vi "Compute Process Data.vi"(0 "Acquisition mode":T1, 5 "Processing loop variables":T3 {"CurrInverter"."last updated" format="%<%H:%M\n%d/%m/%Y>T"; "CurrInverter"."set flag" items=["False", "True"]}, 7 "InverterWaveforms":T11, 9 "ESR scaling":T10[](array[typedef]), 11 "error in (no error)":errorcluster, 12 "Use dummy Vout?":bool, 13 "Dummy Vrms":dbl=120.0, 14 "reset averaging":bool) -> (4 "DataProcAuxData":T2[](array[typedef]), 6 "Processing loop vars out":T3 {"CurrInverter"."last updated" format="%<%H:%M\n%d/%m/%Y>T"; "CurrInverter"."set flag" items=["False", "True"]}, 8 "Max ESR":dbl[](array[numeric]), 15 "error out":errorcluster)   [LabVIEW 2019, in "Main.lvclass"]
doc: "Developed by Kevin Thompson\nkevin@thompsonengineering.net\n\nCopyright 2020\nThompson Engineering, LLC"
uses:
  Main.lvclass
  subvis/DataTypes/Processing loop variables--cluster.ctl
  subvis/DataTypes/averaging variables.ctl
  subvis/DataTypes/ESR alarm variables.ctl
  Common/DataTypes/Inverter database record v2--cluster.ctl
  Common/DataTypes/inverter info v2--cluster.ctl
  Common/DataTypes/inverter gain range--cluster.ctl
  Common/DataTypes/inverter offset range--cluster.ctl
  Common/DataTypes/InverterWaveforms--cluster.ctl
  Common/DataTypes/ChannelWaveforms--cluster.ctl
  subvis/DataTypes/ESR scaling--cluster.ctl
  DataTypes/DataProcessAuxData--cluster.ctl
  Common/DataTypes/Acquisition Mode--cluster.ctl
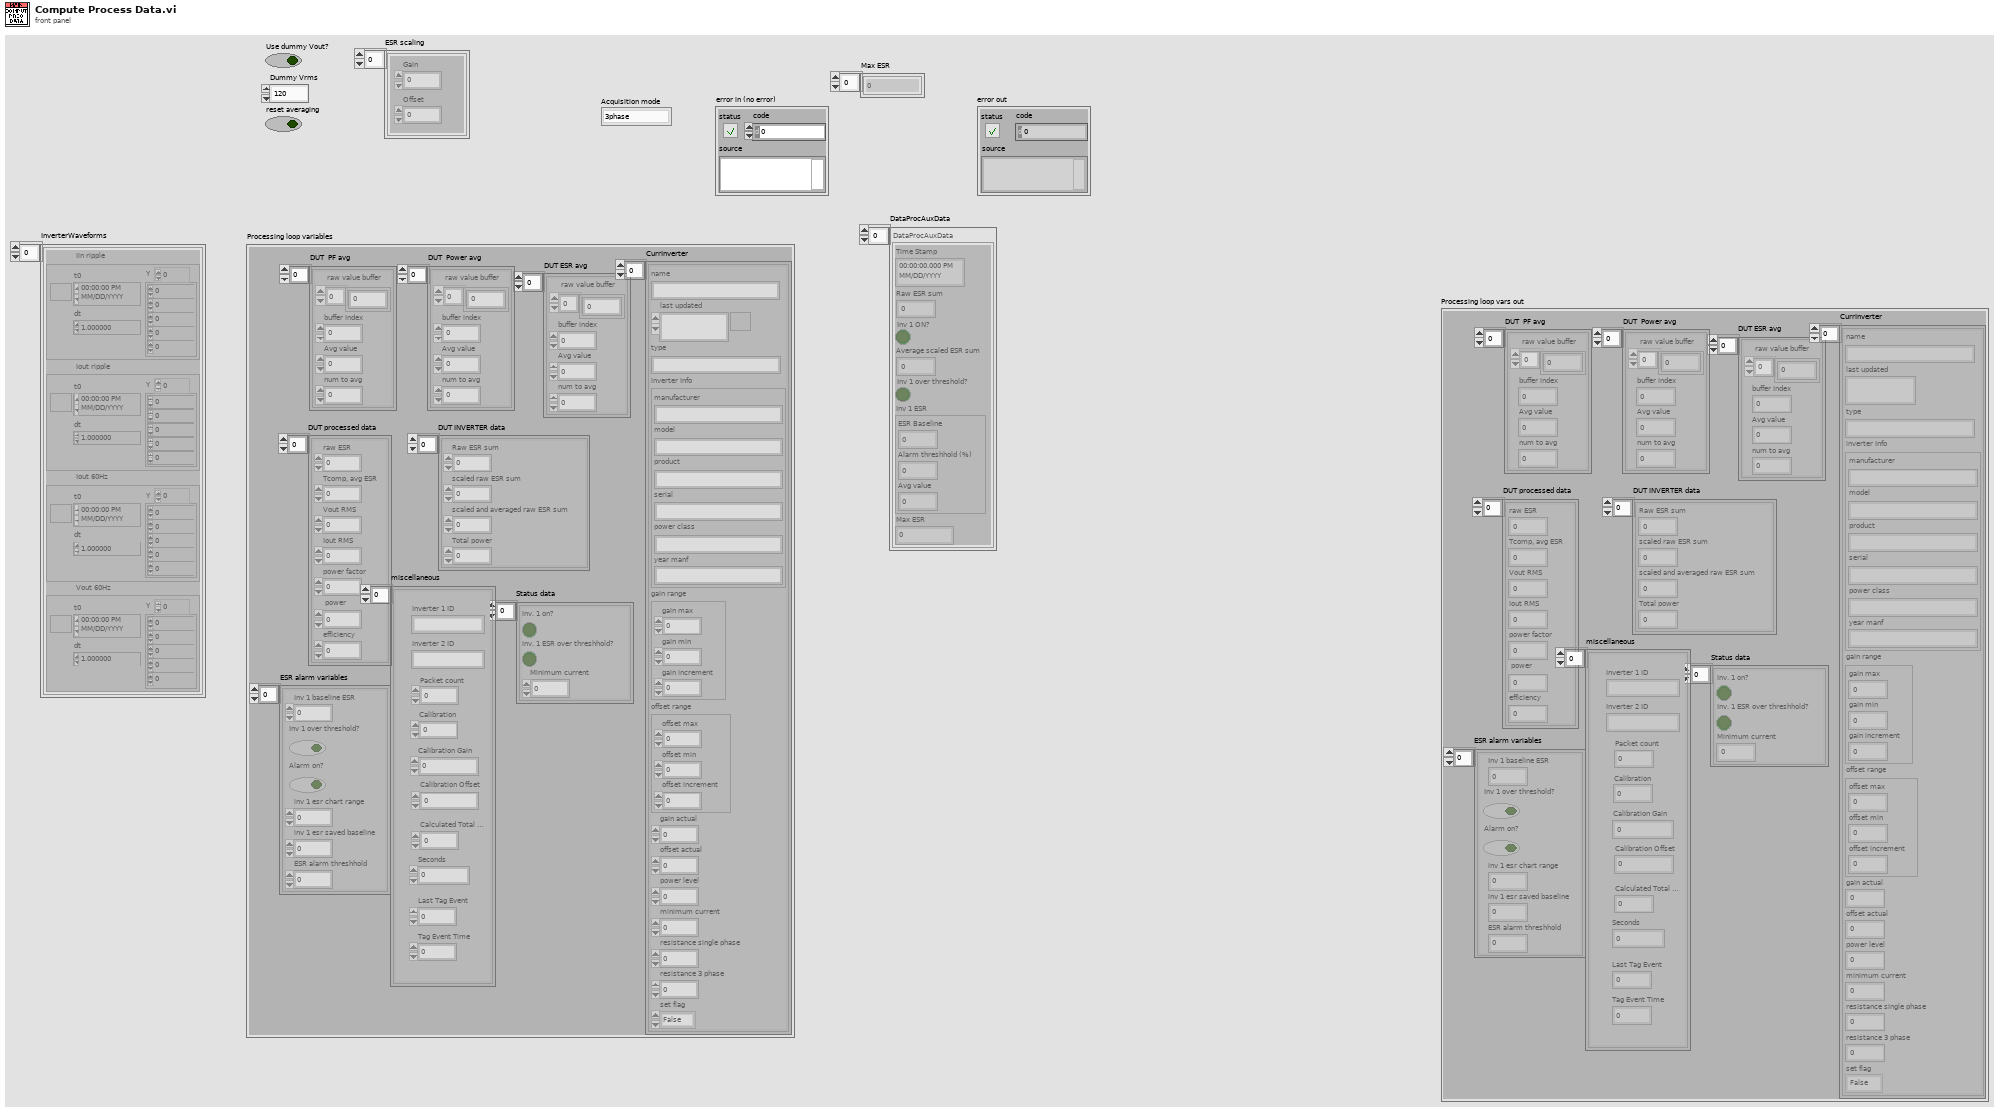
[diagram p1: front panel]
types:
  T1 = typedef "Acquisition Mode--cluster.ctl" = enum16{"3phase", "Single"}
  T2 = typedef "DataProcessAuxData--cluster.ctl" = cluster{"Time Stamp":timestamp, "Raw ESR sum":dbl, "Inv 1 ON?":bool, "Average scaled ESR sum":dbl, "Inv 1 over threshold?":bool, "Inv 1 ESR":cluster{"ESR Baseline":dbl, "Alarm threshhold (%)":dbl, "Avg value":dbl}, "Max ESR":dbl}
  T3 = typedef "Main.lvclass/Processing loop variables--cluster.ctl" = cluster{"DUT ESR avg":T4[], "DUT  PF avg":T4[], "DUT  Power avg ":T4[], "DUT processed data":cluster{"raw ESR":dbl, "Tcomp, avg ESR":dbl, "Vout RMS":dbl, "Iout RMS":dbl, "power factor":dbl, "power":dbl, "efficiency":dbl}[], "ESR alarm variables":T5[], "Status data":cluster{"Inv. 1 on?":bool, "Inv. 1 ESR over threshhold?":bool, "Minimum current":dbl}[], "CurrInverter":T6[], "miscellaneous":cluster{"Inverter 1 ID":string, "Inverter 2 ID":string, "Packet count":u32, "Calibration":dbl, "Calibration Gain":dbl, "Calibration Offset":dbl, "Calculated Total Power":dbl, "Seconds":dbl, "Last Tag Event":dbl, "Tag Event Time":dbl}[], "DUT INVERTER data":cluster{"Raw ESR sum":dbl, "scaled raw ESR sum":dbl, "scaled and averaged raw ESR sum":dbl, "Total power":dbl}[]}
  T4 = typedef "Main.lvclass/averaging variables.ctl" = cluster{"raw value buffer":dbl[], "buffer index":i32, "Avg value":dbl, "num to avg":i32}
  T5 = typedef "Main.lvclass/ESR alarm variables.ctl" = cluster{"Inv 1 baseline ESR":dbl, "Inv 1 over threshold?":bool, "Alarm on?":bool, "inv 1 esr chart range":dbl, "inv 1 esr saved baseline":dbl, "ESR alarm threshhold":dbl}
  T6 = typedef "Inverter database record v2--cluster.ctl" = cluster{"name":string, "last updated":timestamp, "type":string, "inverter Info":T7, "gain range":T8, "offset range":T9, "gain actual":dbl, "offset actual":dbl, "power level":dbl, "minimum current":dbl, "resistance single phase":dbl, "resistance 3 phase":dbl, "set flag":u16}
  T7 = typedef "inverter info v2--cluster.ctl" = cluster{"manufacturer":string, "model":string, "product":string, "serial":string, "power class":string, "year manf":string}
  T8 = typedef "inverter gain range--cluster.ctl" = cluster{"gain max":dbl, "gain min":dbl, "gain increment":dbl}
  T9 = typedef "inverter offset range--cluster.ctl" = cluster{"offset max":dbl, "offset min":dbl, "offset increment":dbl}
  T10 = typedef "Main.lvclass/ESR scaling--cluster.ctl" = cluster{"Gain":dbl, "Offset":dbl}
  T11 = typedef "InverterWaveforms--cluster.ctl" = T12[]
  T12 = typedef "ChannelWaveforms--cluster.ctl" = cluster{"Iin ripple ":waveform(dbl), "Iout ripple ":waveform(dbl), "Iout 60Hz":waveform(dbl), "Vout 60Hz":waveform(dbl)}
  T13 = cluster{"ESR Baseline":dbl, "Alarm threshhold (%)":dbl, "Avg value":dbl}[]
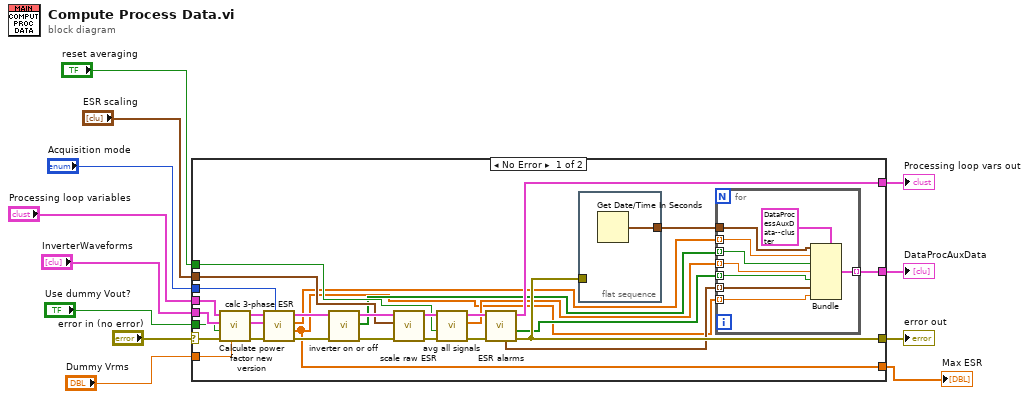
[diagram p0: block diagram]
diagram:
  n1 = case shown="No Error" "error in (no error)" {
    selector: "error in (no error)" -> [w23 w53]
    tunnel: "Processing loop variables" -> [w41 w52]
    tunnel: "InverterWaveforms" -> [w40 _]
    tunnel: "Use dummy Vout?" -> [w39 _]
    tunnel: "Dummy Vrms" -> [w38 _]
    tunnel: "ESR scaling" -> [w30 _]
    tunnel: "reset averaging" -> [w28 _]
    tunnel: [w24 w52] -> w6
    tunnel: [w20 w53] -> w4
    tunnel: [w22 _] -> w3
    tunnel: "Acquisition mode" -> [w19 _]
    tunnel: [w13 _] -> w1
    frame No Error {
      n2 = call "Calculate power factor new version.vi"("Dummy Vrms"=w38, "error in"=w23, "Use dummy Vout?"=w39, "InverterWaveforms"=w40, "Processing loop variables"=w41) -> ("error out"=w37:errorcluster, "InverterWaveforms"=w36:T11, "Processing loop variables out"=w35:T3)  [unwired: 3 in]
      n3 = call "calc 3-phase ESR.vi"("Acquisition mode"=w19, "error in"=w37, "InverterWaveforms"=w36, "Processing loop variables"=w35) -> ("error out"=w34:errorcluster, "Max ESR"=w13:dbl[], "Raw ESR sum"=w18:dbl[], "Processing loop variables"=w33:T3)  [unwired: 4 in]
      n4 = call "inverter on or off.vi"("error in (no error)"=w34, "Processing loop variables"=w33) -> ("error out"=w31:errorcluster, "Inv 1 ON?"=w17:bool[], "processing loop vars out"=w32:T3)  [unwired: 7 in]
      n5 = call "scale raw ESR.vi"("error in (no error)"=w31, "ESR scaling"=w30, "Processing loop variables"=w32) -> ("error out"=w27:errorcluster, "Processing loop variables out"=w29:T3)  [unwired: 7 in]
      n6 = call "avg all signals.vi"("error in (no error)"=w27, "reset averaging"=w28, "processing loop vars"=w29) -> ("error out"=w25:errorcluster, "Average scaled ESR sum"=w14:dbl[], "processing loop vars out"=w26:T3)  [unwired: 5 in]
      n7 = call "ESR alarms.vi"("error in (no error)"=w25, "Processing loop variables"=w26) -> ("error out"=w20:errorcluster, "Inv 1 over threshold?"=w15:bool[], "Processing loop vars out"=w24:T3, "Inv 1 ESR"=w16:T13)  [unwired: 6 in]
      n8 = flat-sequence {
        tunnel: [w51] -> w21
        tunnel: w20 -> [_]
        frame #0 {
          n9 = Get Date/Time In Seconds() -> (seconds since 1Jan1904=w51:timestamp)
        }
      }
      n10 = for {
        tunnel: [w50] -> w22 mode=indexing
        tunnel: w21 -> [w48]
        tunnel: w13 -> [w47] mode=indexing
        tunnel: w18 -> [w46] mode=indexing
        tunnel: w17 -> [w45] mode=indexing
        tunnel: w14 -> [w44] mode=indexing
        tunnel: w16 -> [w43] mode=indexing
        tunnel: w15 -> [w42] mode=indexing
        n11 = Bundle(cluster=T2 {"Time Stamp"=timestamp(0 s since 1904-01-01), "Raw ESR sum"=0.0, "Inv 1 ON?"=FALSE, "Average scaled ESR sum"=0.0, "Inv 1 over threshold?"=FALSE, "Inv 1 ESR"={"ESR Baseline"=0.0, "Alarm threshhold (%)"=0.0, "Avg value"=0.0}, "Max ESR"=0.0} ("DataProcAuxData"), "Time Stamp"=w48, "Raw ESR sum"=w46, "Inv 1 ON?"=w45, "Average scaled ESR sum"=w44, "Inv 1 over threshold?"=w42, "Inv 1 ESR"=w43, "Max ESR"=w47) -> (w50:T2)
      }
    }
    frame Error {
    }
  }
  "error out" <- w4
  "Processing loop vars out" <- w6
  "DataProcAuxData" <- w3
  "Max ESR" <- w1
